vi "翻转01.vi"(1 "收到的信息序列":i32[](array[numeric])) -> (0 "翻转后的波形":i32[](array[numeric]))   [LabVIEW 2013]
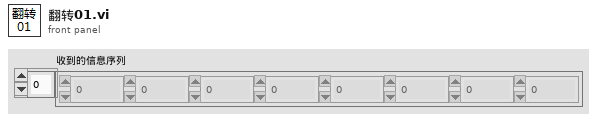
[diagram p1: front panel]
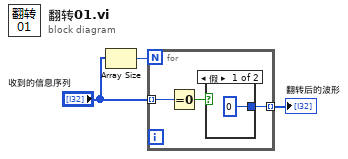
[diagram p0: block diagram]
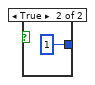
[diagram p2: hidden frame]
diagram:
  n1 = Array Size(array="收到的信息序列") -> (size(s)=w3:i32)
  n2 = for {
    N: w3 -> [_]
    tunnel: "收到的信息序列" -> [w6] mode=indexing
    tunnel: [w4] -> w1 mode=indexing
    n3 = Equal To 0?(x=w6) -> (x = 0?=w5:bool)
    n4 = case shown="假" w5 {
      tunnel: [0 1] -> w4
      frame False {
      }
      frame True {
      }
    }
  }
  "翻转后的波形" <- w1
